vi "Address Claim Address.vi"(8 "error in":errorcluster, 9 "Byte Cluster":u8[](array[numeric]), 10 "Requested Address":u8, 11 "Write Session":refnum<k21>) -> (0 "error out":errorcluster, 3 "Write Session out":refnum<k21>)   [LabVIEW 2013, in "J1939 Addon Engine.lvlib"]
uses:
  Engine/J1939 Addon Engine.lvlib
  J1939 Utilities/Types/CAN Outgoing Message Cluster.ctl
  J1939 Utilities/Types/PGN Fields Cluster.ctl
  J1939 Utilities/SubVIs/Convert J1939 ID to CAN Arb ID.vi
  <vilib>/xnet/xnet.llb/XNET Write (Frame CAN).vi
  J1939 Utilities/J1939 Utilities.lvlib
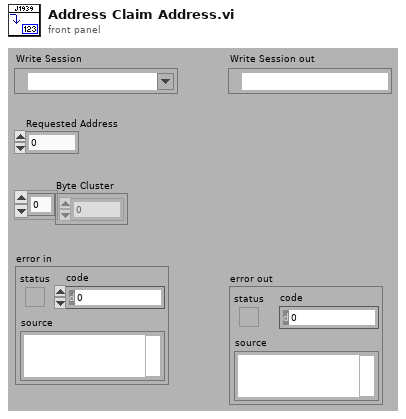
[diagram p1: front panel]
types:
  T1 = typedef "J1939 Utilities.lvlib/PGN Fields Cluster.ctl" = cluster{"Reserved Bit":u8, "Data page":u8, "PDU Format":u8, "PDU Specific":u8}
  T2 = typedef "J1939 Utilities.lvlib/CAN Outgoing Message Cluster.ctl" = cluster{"Identifier":u32, "Data":u8[]}
  T3 = typedef "XNET Frame CAN.ctl" = cluster{"timestamp":timestamp, "payload":u8[], "identifier":u32, "type":T4, "extended?":bool, "echo?":bool}
  T4 = typedef "XNET Frame Type CAN.ctl" = u8
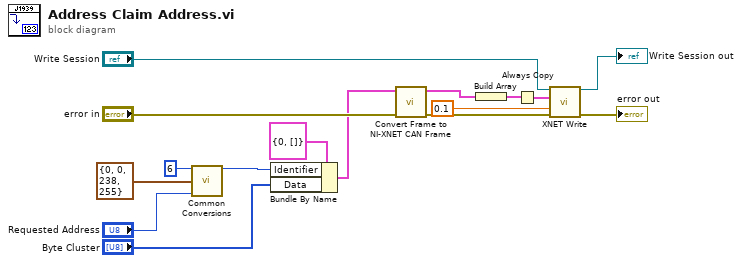
[diagram p0: block diagram]
diagram:
  n1 = call-poly "Common Conversions.vi"("Priority"=u8 6, "PGN Fields"=T1 {"Reserved Bit"=0, "Data page"=0, "PDU Format"=238, "PDU Specific"=255}, "Source Address"="Requested Address") -> ("ID"=w15:u32)  [unwired: 2 in, 10 out]
  n2 = Bundle By Name(cluster=T2 {"Identifier"=0, "Data"=[]} ("Data to Send"), "Identifier"=w15, "Data"="Byte Cluster") -> (w5:T2)
  n3 = call "Convert Frame to NI-XNET CAN Frame.vi"("error in (no error)"="error in", "Data to Send"=w5) -> ("error out"=w6:errorcluster, "CAN frame"=w11:T3)  [unwired: 8 in]
  n4 = Build Array(w11) -> (w2:T3[])
  n5 = Always Copy(1:w2) -> (0:w1:T3[])
  n6 = call-poly <vilib>:"XNET Write.vi"("session in"="Write Session", "data"=w1, "timeout (10)"=0.1, "error in (no error)"=w6) -> ("session out"=→"Write Session out":refnum<k21>, "error out"=→"error out":errorcluster)  [unwired: 10 out]
